vi "FW Get Position Actual.vi"(0 "Notifier Name In":string, 2 "Wait for Finish":bool=TRUE, 11 "Error In":errorcluster) -> (4 "Notifier Name Out":string, 8 "Actual Position":i32, 15 "Error Out":errorcluster)   [LabVIEW 2020]
uses:
  FW Type Defs/FW Notifier Type.ctl
  FW Type Defs/FW Actions.ctl
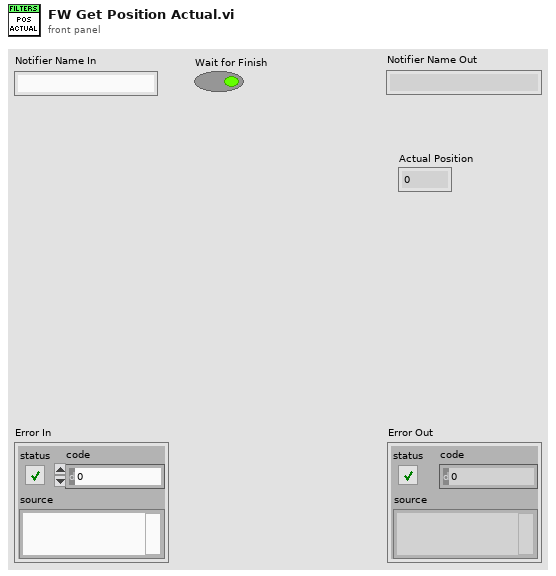
[diagram p1: front panel]
types:
  T1 = typedef "FW Notifier Type.ctl" = cluster{"Actions":T2, "Set Position":u8, "Actual Position":u8, "Speed":dbl, "Num Positions":u8, "Received":bool}
  T2 = typedef "FW Actions.ctl" = enum16{"Set Position", "Get Position", "Get Num Positions", "Set Speed", "Confirm Pos", "Quit"}
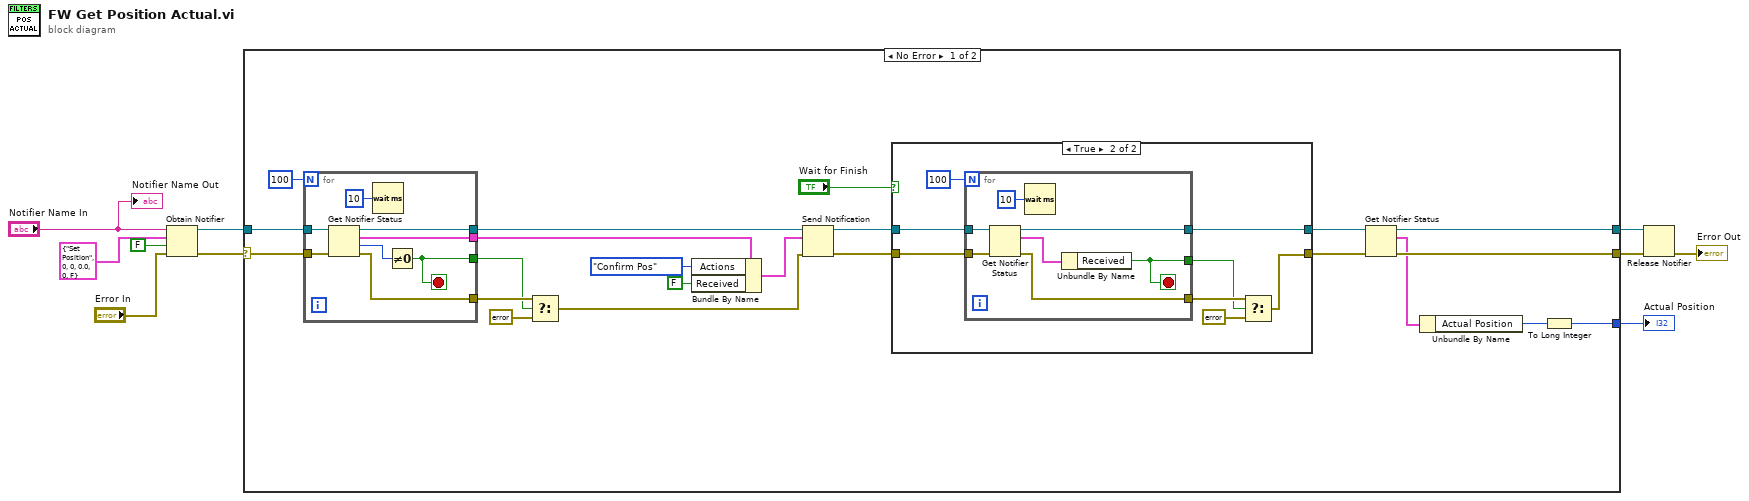
[diagram p0: block diagram]
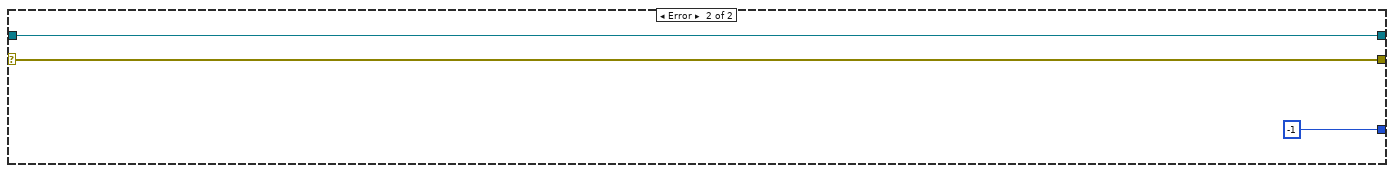
[diagram p3: hidden frame]
diagram:
  n1 = Obtain Notifier(name (unnamed)="Notifier Name In", notification data type=T1 {"Actions"=enum."Set Position", "Set Position"=0, "Actual Position"=0, "Speed"=0.0, "Num Positions"=0, "Received"=FALSE} ("FW102C Note Type"), create if not found? (T)=FALSE, error in (no error)="Error In") -> (notifier out=w7:refnum<notifier>, error out=w8:errorcluster)  [unwired: 1 out]
  n2 = case shown="No Error" w8 {
    selector: w8 -> [w30 w60]
    tunnel: w7 -> [w32 w59]
    tunnel: [w15 w60] -> w4
    tunnel: [w16 w59] -> w5
    tunnel: [w12 -1 ("Actual Position")] -> w1
    frame No Error {
      n3 = for {
        N: 100 -> [_]
        tunnel: w32 -> [w57]
        tunnel: [w55] -> w23
        tunnel: [w53] -> w29
        tunnel: w30 -> [w52]
        tunnel: [w51] -> w24
        tunnel: [w50] -> w19
        stop <- w55 stop-if-true
        n4 = Get Notifier Status(notifier=w57, error in (no error)=w52) -> (notifier out=w53:refnum<notifier>, current notification=w50:T1, # waiting=w56:i32, error out=w51:errorcluster)  [unwired: 1 out]
        n5 = Wait (ms)(milliseconds to wait=u32 10) -> ()  [unwired: 1 out]
        n6 = Not Equal To 0?(x=w56) -> (x != 0?=w55:bool)
      }
      n7 = Select(t=w24, s=w23, f=errorcluster {"status"=TRUE, "code"=0, "source"="Filter wheel busy. Timeout error."}) -> (s? t:f=w11:errorcluster)
      n8 = Bundle By Name(cluster=w19, "Actions"=FW_Actions."Confirm Pos", "Received"=FALSE) -> (w28:T1)
      n9 = Send Notification(notification=w28, notifier=w29, error in (no error)=w11) -> (notifier out=w26:refnum<notifier>, error out=w27:errorcluster)
      n10 = case shown="True" "Wait for Finish" {
        tunnel: w27 -> [w33 w42]
        tunnel: w26 -> [w34 w41]
        tunnel: [w34 w40] -> w18
        tunnel: [w33 w39] -> w17
        frame False {
        }
        frame True {
          n11 = for {
            N: 100 -> [_]
            tunnel: w41 -> [w49]
            tunnel: [w47] -> w40
            tunnel: w42 -> [w46]
            tunnel: [w45] -> w37
            tunnel: [w43] -> w36
            stop <- w43 stop-if-true
            n12 = Get Notifier Status(notifier=w49, error in (no error)=w46) -> (notifier out=w47:refnum<notifier>, current notification=w44:T1, error out=w45:errorcluster)  [unwired: 2 out]
            n13 = Wait (ms)(milliseconds to wait=u32 10) -> ()  [unwired: 1 out]
            n14 = Unbundle By Name(w44) -> ("Received"=w43:bool)
          }
          n15 = Select(t=w37, s=w36, f=errorcluster {"status"=TRUE, "code"=0, "source"="Filter Wheel Error: Action didn't complete."}) -> (s? t:f=w39:errorcluster)
        }
      }
      n16 = Get Notifier Status(notifier=w18, error in (no error)=w17) -> (notifier out=w16:refnum<notifier>, current notification=w14:T1, error out=w15:errorcluster)  [unwired: 2 out]
      n17 = Unbundle By Name(w14) -> ("Actual Position"=w13:u8)
      n18 = To Long Integer(number=w13) -> (32bit integer=w12:i32)
    }
    frame Error {
    }
  }
  "Actual Position" <- w1
  n19 = Release Notifier(notifier=w5, error in (no error)=w4) -> (error out=→"Error Out":errorcluster)  [unwired: 1 in, 2 out]
  "Notifier Name Out" <- "Notifier Name In"
